vi "Parse Label.vi"(8 "error in":errorcluster, 9 "channel #":u16, 10 "direction":string, 11 "node in":refnum<k20>) -> (0 "error out":errorcluster, 3 "labels":T1[](array[typedef]) {"Label (octal)" format="%o"})   [LabVIEW 2020, in "ARINC 429 Import.lvlib"]
uses:
  ARINC 429 Import.lvlib
  Types/Label.ctl
  Types/Parameter.ctl
  Encoding and Decoding/Encoding.ctl
  <resource>/objmgr/DOMUserDefRef.rc
  <vilib>/xml/NI_XML.lvlib
  Encoding and Decoding/Encoding and Decoding.lvlib
  Read Tag Element (Boolean).vi
  Read Tag Element (String).vi
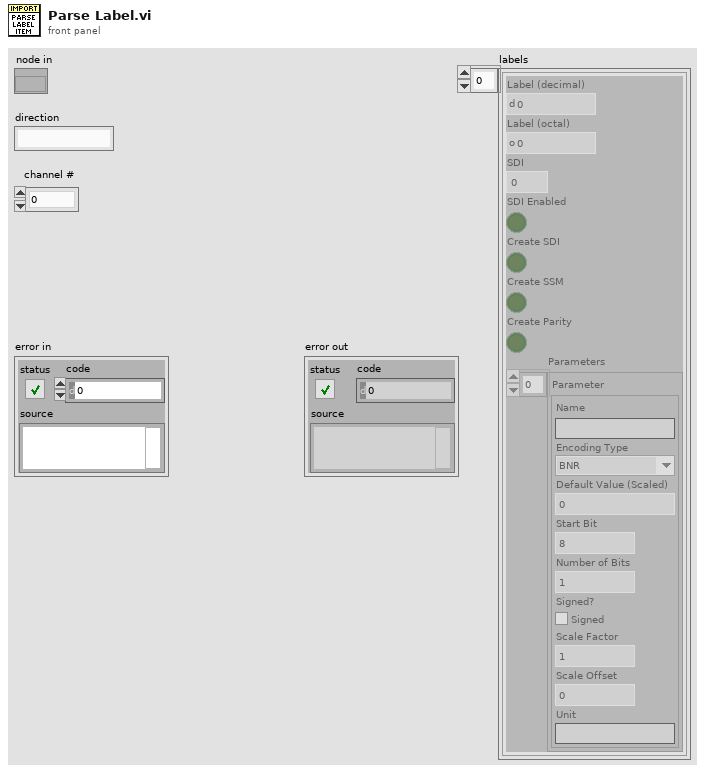
[diagram p1: front panel]
types:
  T1 = typedef "ARINC 429 Import.lvlib/Label.ctl" = cluster{"Label (decimal)":i32, "Label (octal)":i32, "SDI":u8, "SDI Enabled":bool, "Create SDI":bool, "Create SSM":bool, "Create Parity":bool, "Parameters":T2[]}
  T2 = typedef "ARINC 429 Import.lvlib/Parameter.ctl" = cluster{"Name":string, "Encoding Type":T3, "Default Value (Scaled)":dbl, "Start Bit":i32, "Number of Bits":i32, "Signed?":bool, "Scale Factor":dbl, "Scale Offset":dbl, "Unit":string}
  T3 = typedef "Encoding and Decoding.lvlib/Encoding.ctl" = enum16{"BNR", "BCD", "Discrete"}
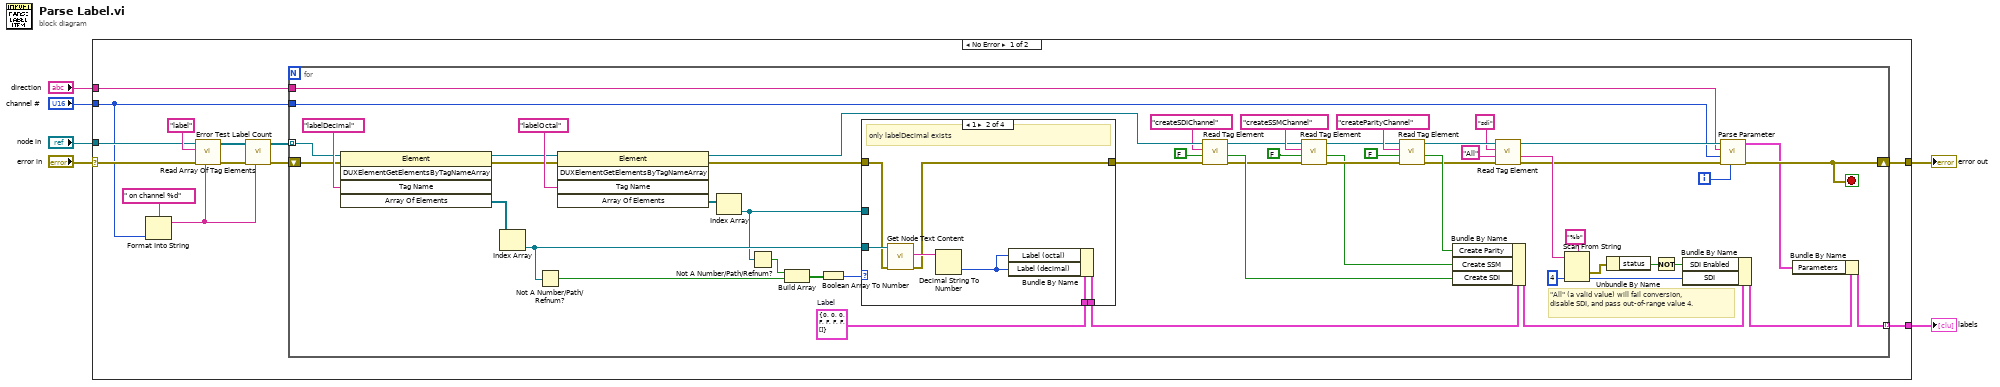
[diagram p0: block diagram]
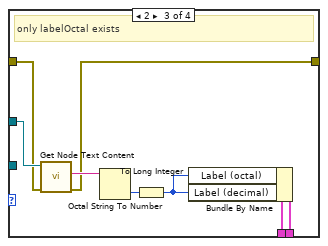
[diagram p3: hidden frame]
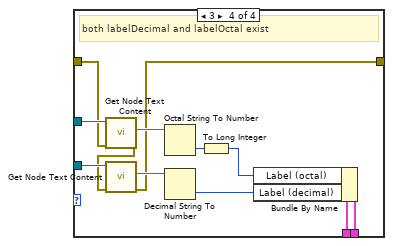
[diagram p4: hidden frame]
diagram:
  n1 = case shown="No Error" "error in" {
    selector: "error in" -> [w10 w102]
    tunnel: [w19 _] -> w6
    tunnel: "node in" -> [w13 _]
    tunnel: [w12 w102] -> w4
    tunnel: "direction" -> [w11 _]
    tunnel: "channel #" -> [w8 _]
    frame No Error {
      n2 = Format Into String(format string=" on channel %d", w8) -> (resulting string=w7:string)  [unwired: 2 in, 1 out]
      n3 = call "Read Array Of Tag Elements.vi"("error text in"=w7, "error in"=w10, "tag name"="label" ("Tag Name"), "node in"=w13) -> ("error out"=w15:errorcluster, "array of elements"=w17:refnum<k20>[])  [unwired: 6 in]
      n4 = call "Error Test Label Count.vi"("error text in"=w7, "error in"=w15, "array of elements"=w17) -> ("error out"=w14:errorcluster, "array of elements out"=w16:refnum<k20>[])  [unwired: 7 in]
      n5 = for {
        shift-right: [w25] -> w12
        shift-left: w14 -> [w71]
        tunnel: [w29] -> w19 mode=indexing
        tunnel: w16 -> [w27] mode=indexing
        tunnel: w11 -> [w22]
        tunnel: w8 -> [w21]
        i -> [w20]
        stop <- w25 stop-if-true
        w28 = T1 {"Label (decimal)"=0, "Label (octal)"=0, "SDI"=0, "SDI Enabled"=FALSE, "Create SDI"=FALSE, "Create SSM"=FALSE, "Create Parity"=FALSE, "Parameters"=[]}  # Label
        # "\"All\" (a valid value) will fail conversion, disable SDI, and pass out-of-range value 4."
        n6 = invoke class="Element" method="DUXElementGetElementsByTagNameArray"(reference=w27, error in=w71, "Tag Name"="labelDecimal") -> (reference out=w67:refnum<k20>, error out=w66:errorcluster, "Array Of Elements"=w70:refnum<k20>[])  [unwired: 2 in, 2 out]
        n7 = Index Array(array=w70) -> (element=w61:refnum<k20>)  [unwired: 1 in]
        n8 = Not A Number/Path/Refnum?(number/path/refnum=w61) -> (NaN/Path/Refnum?=w64:bool)
        n9 = invoke class="Element" method="DUXElementGetElementsByTagNameArray"(reference=w67, error in=w66, "Tag Name"="labelOctal") -> (reference out=w57:refnum<k20>, error out=w59:errorcluster, "Array Of Elements"=w69:refnum<k20>[])  [unwired: 2 in, 2 out]
        n10 = Index Array(array=w69) -> (element=w60:refnum<k20>)  [unwired: 1 in]
        n11 = Not A Number/Path/Refnum?(number/path/refnum=w60) -> (NaN/Path/Refnum?=w65:bool)
        n12 = Build Array(w65, w64) -> (w63:bool[])
        n13 = Boolean Array To Number(Boolean array=w63) -> (number=w62:u32)
        n14 = case shown="1" w62 {
          tunnel: w28 -> [w74 w80 w88 w100]
          tunnel: [w74 w79 w87 w99] -> w56
          tunnel: w61 -> [_ w78 _ w96]
          tunnel: w60 -> [_ _ w85 w97]
          tunnel: w59 -> [w73 w76 w83 w92]
          tunnel: [w73 w75 w82 w90] -> w58
          frame 0, Default {
            # "neither labelDecimal or labelOctal exist"
          }
          frame 1 {
            # "only labelDecimal exists"
            n15 = call <vilib>:"Get Node Text Content.vi"("error in (no error)"=w76, "node in"=w78) -> ("error out"=w75:errorcluster, "node text"=w81:string)  [unwired: 7 in, 1 out]
            n16 = Decimal String To Number(string=w81) -> (number=w77:i32)  [unwired: 2 in, 1 out]
            n17 = Bundle By Name(cluster=w80, "Label (octal)"=w77, "Label (decimal)"=w77) -> (w79:T1)
          }
          frame 2 {
            # "only labelOctal exists"
            n18 = call <vilib>:"Get Node Text Content.vi"("error in (no error)"=w83, "node in"=w85) -> ("error out"=w82:errorcluster, "node text"=w89:string)  [unwired: 7 in, 1 out]
            n19 = Octal String To Number(4:w89) -> (0:w86:u32)  [unwired: 2 in, 1 out]
            n20 = To Long Integer(number=w86) -> (32bit integer=w84:i32)
            n21 = Bundle By Name(cluster=w88, "Label (octal)"=w84, "Label (decimal)"=w84) -> (w87:T1)
          }
          frame 3 {
            # "both labelDecimal and labelOctal exist"
            n22 = call <vilib>:"Get Node Text Content.vi"("error in (no error)"=w92, "node in"=w97) -> ("error out"=w91:errorcluster, "node text"=w98:string)  [unwired: 7 in, 1 out]
            n23 = call <vilib>:"Get Node Text Content.vi"("error in (no error)"=w91, "node in"=w96) -> ("error out"=w90:errorcluster, "node text"=w101:string)  [unwired: 7 in, 1 out]
            n24 = Octal String To Number(4:w98) -> (0:w94:u32)  [unwired: 2 in, 1 out]
            n25 = Decimal String To Number(string=w101) -> (number=w95:i32)  [unwired: 2 in, 1 out]
            n26 = To Long Integer(number=w94) -> (32bit integer=w93:i32)
            n27 = Bundle By Name(cluster=w100, "Label (octal)"=w93, "Label (decimal)"=w95) -> (w99:T1)
          }
        }
        n28 = call-poly "Read Tag Element.vi"("error in"=w58, "default"=FALSE, "Tag Name"="createSDIChannel", "node in"=w57) -> ("error out"=w50:errorcluster, "value"=w54:bool, "node out"=w51:refnum<k20>)  [unwired: 5 in]
        n29 = call-poly "Read Tag Element.vi"("error in"=w50, "default"=FALSE, "Tag Name"="createSSMChannel", "node in"=w51) -> ("error out"=w49:errorcluster, "value"=w47:bool, "node out"=w48:refnum<k20>)  [unwired: 5 in]
        n30 = call-poly "Read Tag Element.vi"("error in"=w49, "default"=FALSE, "Tag Name"="createParityChannel", "node in"=w48) -> ("error out"=w39:errorcluster, "value"=w46:bool, "node out"=w42:refnum<k20>)  [unwired: 5 in]
        n31 = Bundle By Name(cluster=w56, "Create Parity"=w46, "Create SSM"=w47, "Create SDI"=w54) -> (w41:T1)
        n32 = call-poly "Read Tag Element.vi"("error in"=w39, "default"="All", "Tag Name"="sdi", "node in"=w42) -> ("error out"=w26:errorcluster, "value"=w31:string, "node out"=w24:refnum<k20>)  [unwired: 5 in]
        n33 = Scan From String(format string="%b", input string=w31, default 1=u8 4 ("default value 1")) -> (error out=w34:errorcluster, output 1=w35:u8)  [unwired: 2 in, 2 out]
        n34 = Unbundle By Name(w34) -> ("status"=w33:bool)
        n35 = Not(x=w33) -> (.not. x?=w32:bool)
        n36 = Bundle By Name(cluster=w41, "SDI Enabled"=w32, "SDI"=w35) -> (w30:T1)
        n37 = call "Parse Parameter.vi"("label index"=w20, "error in"=w26, "channel #"=w21, "direction"=w22, "node in"=w24) -> ("error out"=w25:errorcluster, "parameters"=w23:T2[])  [unwired: 5 in]
        n38 = Bundle By Name(cluster=w30, "Parameters"=w23) -> (w29:T1)
      }
    }
    frame Error {
    }
  }
  "labels" <- w6
  "error out" <- w4
